vi "Change table column color.vi"(8 "error in (no error)":errorcluster, 9 "At last screw":bool, 10 "Screw No.":dbl, 11 "Table Control 2":refnum<vi>) -> (0 "error out":errorcluster)   [LabVIEW 2017]
uses:
  <vilib>/Utility/miscctls.llb/LVRowAndColumnTypeDef.ctl
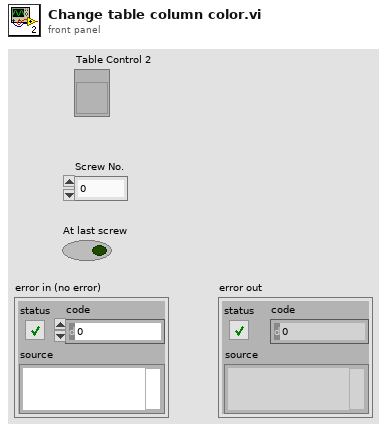
[diagram p1: front panel]
types:
  T1 = typedef "LVRowAndColumnTypeDef.ctl" = cluster{"Row":i32, "Column":i32}
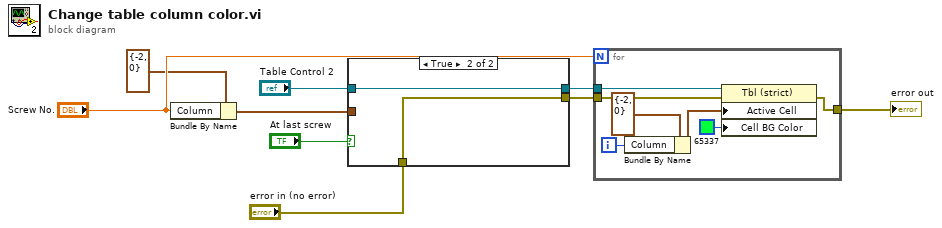
[diagram p0: block diagram]
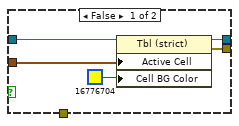
[diagram p2: hidden frame]
diagram:
  n1 = Bundle By Name(cluster=T1 {"Row"=-2, "Column"=0} ("Active Cell:Active Cell"), "Column"="Screw No.") -> (w7:T1)
  n2 = case shown="True" "At last screw" {
    tunnel: w7 -> [w13 _]
    tunnel: [w12 w16] -> w6
    tunnel: [w11 w15] -> w5
    tunnel: "Table Control 2" -> [w10 w16]
    tunnel: "error in (no error)" -> [_ w15]
    frame False {
      n3 = property on="Property Node" class="Tbl (strict)"(reference=w10, "Active Cell"=w13, "Cell BG Color"=u32 16776704) -> (reference out=w12:refnum<vi>, error out=w11:errorcluster)  [unwired: 1 in]
    }
    frame True {
    }
  }
  n4 = for {
    N: "Screw No." -> [_]
    tunnel: w6 -> [w23]
    tunnel: w5 -> [w22]
    tunnel: [w17] -> w2
    i -> [w20]
    n5 = Bundle By Name(cluster=T1 {"Row"=-2, "Column"=0} ("Active Cell:Active Cell"), "Column"=w20) -> (w18:T1)
    n6 = property on="Property Node" class="Tbl (strict)"(reference=w23, error in=w22, "Active Cell"=w18, "Cell BG Color"=u32 65337) -> (error out=w17:errorcluster)  [unwired: 1 out]
  }
  "error out" <- w2
